vi "Test Materials Read and Saving XML.vi"() -> ()   [LabVIEW 2022 SP3]
panel:
  in  "Recipe XML File Path 2":path
  in  "Recipe XML File Path":path=path "X:/Documents/Digilens/Documents/Init files and recipes 04092024/DLP2Initialization.xml"
  in  "Head 1 Material 2":u16(ring) items=["None", "109G", "113A_3", "114A", "507_2", "507_2(50)"]
  in  "Head 2 Material 2":u16(ring) items=["None", "109G", "113A_3", "114A", "507_2", "507_2(50)"]
  in  "Head 3 Material 2":u16(ring) items=["None", "109G", "113A_3", "114A", "507_2", "507_2(50)"]
  in  "Head 4 Material 2":u16(ring) items=["None", "109G", "113A_3", "114A", "507_2", "507_2(50)"]
  in  "Head 5 Material 2":u16(ring) items=["None", "109G", "113A_3", "114A", "507_2", "507_2(50)"]
  in  "Head 6 Material 2":u16(ring) items=["None", "109G", "113A_3", "114A", "507_2", "507_2(50)"]
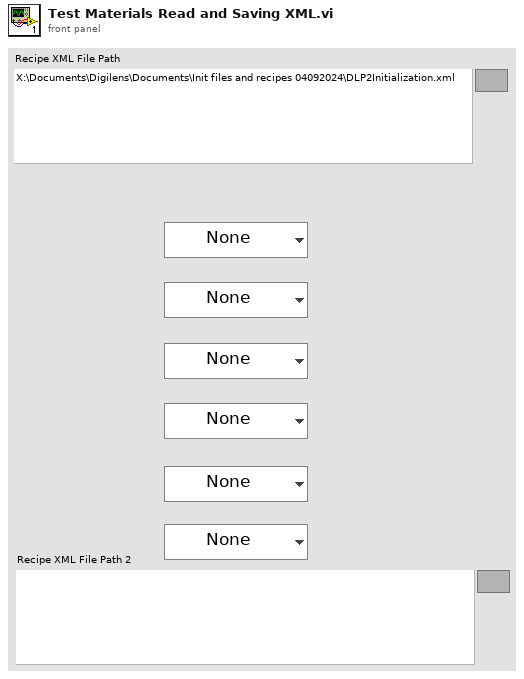
[diagram p1: front panel]
types:
  T1 = typedef "DLPConfig_Initialization.ctl" = cluster{"PrinterInitialization":cluster{"Printer":cluster{"#attributes":cluster{"Name":string}}, "VacPumpSet":cluster{"#attributes":cluster{"VacPumpEnable":bool, "VacPumpSpeed":dbl}}, "HIBEnable":cluster{"#attributes":cluster{"HIB1Enable":bool, "HIB2Enable":bool, "HIB3Enable":bool, "HIB4Enable":bool, "HIB5Enable":bool, "HIB6Enable":bool}}, "PrinterCompensation":T2}, "HeadSet":cluster{"HeadProperties":T3[]}, "InkSet":cluster{"Ink":T5[]}, "Troubleshooting":cluster{"PMBLogging":cluster{"#attributes":cluster{"PMBMonitorDuringPrint":bool, "PMBMonitorDuringIdle":bool, "LogSwatheInputData":bool, "LogSwatheOutputData":bool, "LogPrintheadColourPlanes":bool, "LogPMBCommunication":bool, "LogSimulatedOutput":bool, "LogAllPMBCommunicationData":bool, "LogPMBSpace":bool, "ExtendedPMBSpaceLogging":bool, "LogPMBWriteSpeed":bool, "LogUsbRetries":bool}}, "HIBLogging":cluster{"#attributes":cluster{"HIBMonitoringDuringPrint":bool, "HIBMonitoringLog":bool}}}}
  T2 = typedef "DLP2_PrinterCompensationProperties.ctl" = cluster{"#attributes":cluster{"AppName":string, "PrintWeightMultiplier":dbl, "Rotation":bool, "Driver":string, "Server":string, "Database":string, "User":string, "Password":string}}
  T3 = typedef "DLP2_PrinterHeadProperties.ctl" = cluster{"#attributes":T4}
  T4 = typedef "DLPConfig)Init_HeadPropertyAttr--Cluster.ctl" = cluster{"HeadNumber":u8, "Material":string, "HeadLocalX":dbl, "HeadLocalY":dbl, "HeadRotationAngle":dbl, "VH2L_Hi":dbl, "VH2R_Hi":dbl, "VH1LA_Hi":dbl, "VH1LB_Hi":dbl, "VH1RA_Hi":dbl, "VH1RB_Hi":dbl, "VH2L_Lo":dbl, "VH2R_Lo":dbl, "VH1LA_Lo":dbl, "VH1LB_Lo":dbl, "VH1RA_Lo":dbl, "VH1RB_Lo":dbl}
  T5 = typedef "DLP2_PrinterMaterialProperties.ctl" = cluster{"#attributes":cluster{"InkType":string, "ColorPlane":string, "Heat":dbl, "Meniscus":dbl, "Recirculation":dbl, "PrePrintPurge":bool, "PurgeTime":dbl, "PurgeCount":i32, "Density":dbl, "NumberofDrops":i32, "PrintWeight":dbl}}
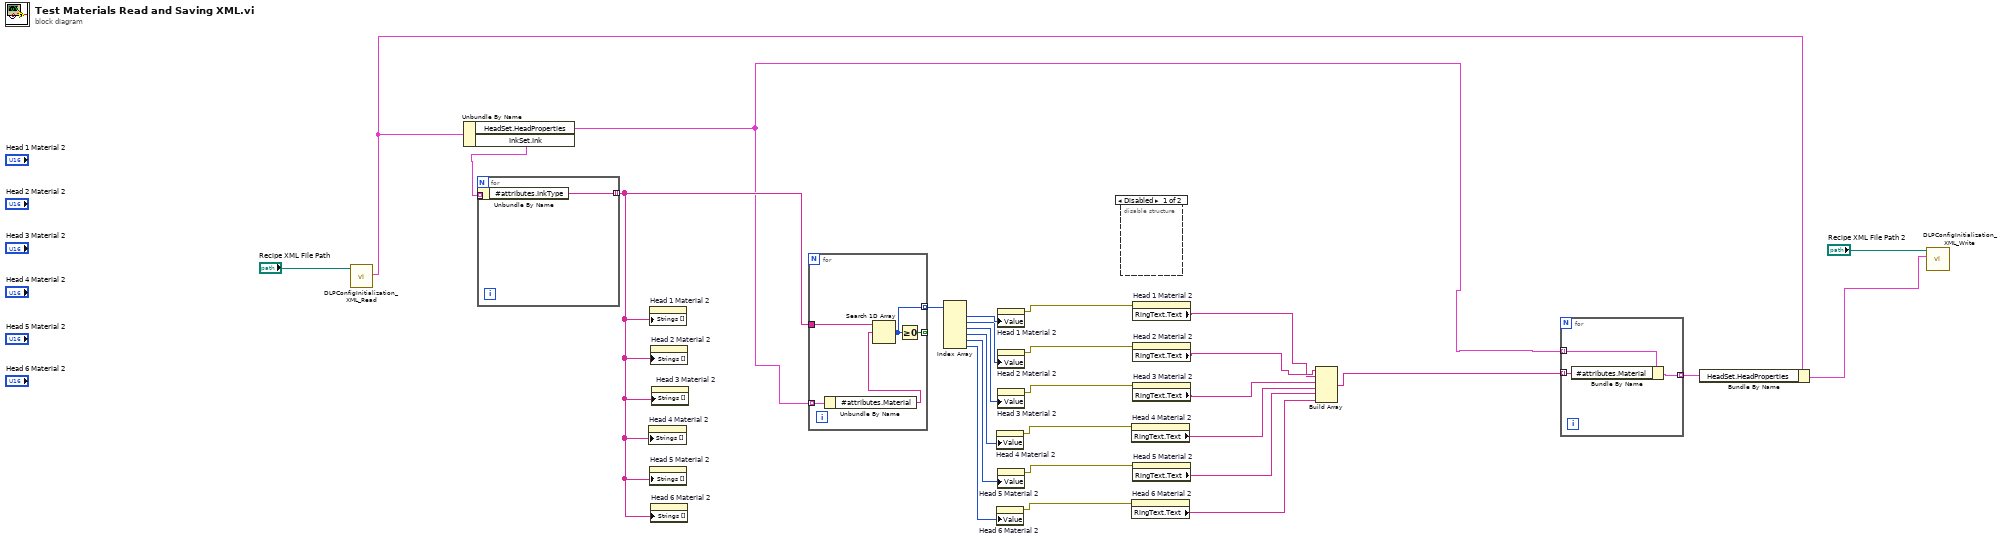
[diagram p0: block diagram]
diagram:
  n1 = call "DLPConfigInitialization_XML_Read.vi"("Recipe XML File Path"="Recipe XML File Path") -> ("DLP"=w4:T1)  [unwired: 9 in, 1 out]
  n2 = Unbundle By Name(w4) -> ("HeadSet.HeadProperties"=w5:T3[], "InkSet.Ink"=w28:T5[])
  n3 = for {
    tunnel: w28 -> [w30] mode=indexing
    tunnel: [w29] -> w25 mode=indexing
    n4 = Unbundle By Name(w30) -> ("#attributes.InkType"=w29:string)
  }
  n5 = property on="Head 4 Material 2" class="Ring (strict)"("Strings []"=w25) -> ()  [unwired: 2 in, 2 out]
  n6 = property on="Head 1 Material 2" class="Ring (strict)"("Strings []"=w25) -> ()  [unwired: 2 in, 2 out]
  n7 = property on="Head 5 Material 2" class="Ring (strict)"("Strings []"=w25) -> ()  [unwired: 2 in, 2 out]
  n8 = property on="Head 2 Material 2" class="Ring (strict)"("Strings []"=w25) -> ()  [unwired: 2 in, 2 out]
  n9 = property on="Head 6 Material 2" class="Ring (strict)"("Strings []"=w25) -> ()  [unwired: 2 in, 2 out]
  n10 = property on="Head 3 Material 2" class="Ring (strict)"("Strings []"=w25) -> ()  [unwired: 2 in, 2 out]
  n11 = for {
    tunnel: w25 -> [w35]
    tunnel: [w33] -> _ mode=indexing
    tunnel: [w32] -> w24 mode=indexing
    tunnel: w5 -> [w31] mode=indexing
    n12 = Unbundle By Name(w31) -> ("#attributes.Material"=w34:string)
    n13 = Search 1D Array(1D array=w35, element=w34) -> (index of element=w32:i32)  [unwired: 1 in]
    n14 = Greater Or Equal To 0?(x=w32) -> (x >= 0?=w33:bool)
  }
  n15 = Index Array(array=w24) -> (element #1=w23:i32, element #2=w22:i32, element #3=w21:i32, element #4=w20:i32, element #5=w19:i32, element #6=w18:i32)  [unwired: 6 in]
  n16 = property on="Head 4 Material 2" class="Ring (strict)"("Value"=w20) -> (error out=w8:errorcluster)  [unwired: 2 in, 1 out]
  n17 = property on="Head 6 Material 2" class="Ring (strict)"("Value"=w18) -> (error out=w10:errorcluster)  [unwired: 2 in, 1 out]
  n18 = property on="Head 1 Material 2" class="Ring (strict)"("Value"=w23) -> (error out=w11:errorcluster)  [unwired: 2 in, 1 out]
  n19 = property on="Head 2 Material 2" class="Ring (strict)"("Value"=w22) -> (error out=w6:errorcluster)  [unwired: 2 in, 1 out]
  n20 = property on="Head 3 Material 2" class="Ring (strict)"("Value"=w21) -> (error out=w7:errorcluster)  [unwired: 2 in, 1 out]
  n21 = property on="Head 5 Material 2" class="Ring (strict)"("Value"=w19) -> (error out=w9:errorcluster)  [unwired: 2 in, 1 out]
  n22 = disable-structure shown="Disabled" {
    frame Disabled {
    }
    frame Enabled {
    }
  }
  n23 = property on="Head 4 Material 2" class="Ring (strict)"(error in=w8) -> ("RingText.Text"=w15:string)  [unwired: 1 in, 2 out]
  n24 = property on="Head 6 Material 2" class="Ring (strict)"(error in=w10) -> ("RingText.Text"=w13:string)  [unwired: 1 in, 2 out]
  n25 = property on="Head 1 Material 2" class="Ring (strict)"(error in=w11) -> ("RingText.Text"=w1:string)  [unwired: 1 in, 2 out]
  n26 = property on="Head 2 Material 2" class="Ring (strict)"(error in=w6) -> ("RingText.Text"=w2:string)  [unwired: 1 in, 2 out]
  n27 = property on="Head 3 Material 2" class="Ring (strict)"(error in=w7) -> ("RingText.Text"=w16:string)  [unwired: 1 in, 2 out]
  n28 = property on="Head 5 Material 2" class="Ring (strict)"(error in=w9) -> ("RingText.Text"=w14:string)  [unwired: 1 in, 2 out]
  n29 = Build Array(w2, w1, w16, w15, w14, w13) -> (w12:string[])
  n30 = for {
    tunnel: w5 -> [w38] mode=indexing
    tunnel: [w37] -> w17 mode=indexing
    tunnel: w12 -> [w36] mode=indexing
    n31 = Bundle By Name(cluster=w38, "#attributes.Material"=w36) -> (w37:T3)
  }
  n32 = Bundle By Name(cluster=w4, "HeadSet.HeadProperties"=w17) -> (w3:T1)
  n33 = call "DLPConfigInitialization_XML_Write.vi"("DLP"=w3, "Recipe XML File Path"="Recipe XML File Path 2") -> ()  [unwired: 9 in, 1 out]
